vi "Drag Panel-Get Window ID.vi"(8 "error in":errorcluster, 10 "Parent Window Handle":u32, 11 "Window Name":string) -> (0 "error out":errorcluster, 3 "Window ID":u32)   [LabVIEW 2018]
uses:
  USER32.DLL
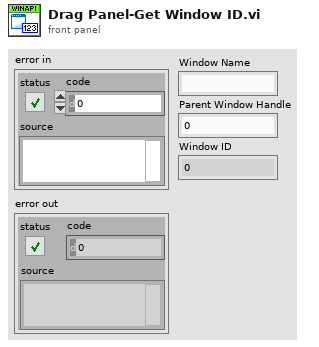
[diagram p1: front panel]
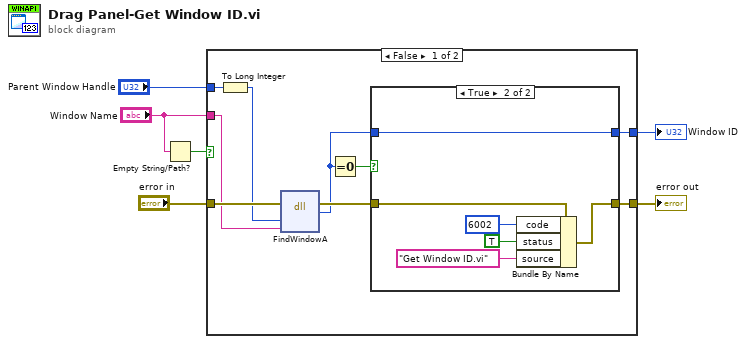
[diagram p0: block diagram]
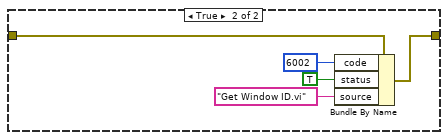
[diagram p3: hidden frame]
diagram:
  n1 = Empty String/Path?(string/path="Window Name") -> (empty?=w5:bool)
  n2 = case shown="False" w5 {
    tunnel: "error in" -> [w15 w25]
    tunnel: "Window Name" -> [w14 _]
    tunnel: "Parent Window Handle" -> [w13 _]
    tunnel: [w8 w24] -> w2
    tunnel: [w7 _] -> w1
    frame False {
      n3 = To Long Integer(number=w13) -> (32bit integer=w12:i32)
      n4 = dll-call lib="user32.dll" fn="FindWindowA"(error in=w15, "lpszClassName"=w12, "lpszWindowName"=w14) -> (error out=w10:errorcluster, "hWnd"=w9:u32)  [unwired: 4 in, 1 out]
      n5 = Equal To 0?(x=w9) -> (x = 0?=w11:bool)
      n6 = case shown="True" w11 {
        tunnel: w10 -> [w17 w23]
        tunnel: w9 -> [w16 w18]
        tunnel: [w17 w19] -> w8
        tunnel: [w16 w18] -> w7
        frame False {
        }
        frame True {
          n7 = Bundle By Name(cluster=w23, "code"=6002, "status"=TRUE, "source"="Get Window ID.vi") -> (w19:errorcluster)
        }
      }
    }
    frame True {
      n8 = Bundle By Name(cluster=w25, "code"=6002, "status"=TRUE, "source"="Get Window ID.vi") -> (w24:errorcluster)
    }
  }
  "error out" <- w2
  "Window ID" <- w1
